vi "CH1603_ONOFF Single Realy.vi"(5 "Loop Read(3)":i32=3, 6 "Relay State":bool, 7 "Device Addr(0x01)":u8=1 format="%02x", 8 "error in (no error)":errorcluster, 9 "Delay Time(200ms)":u32=200, 10 "IO Port No(1~16)":u8=1 format="%02d", 11 "MyIndex":u8) -> (0 "error out":errorcluster, 2 "Result(T:Pass)":bool, 3 "VISA resource name out":refnum<visa-resource-name>)   [LabVIEW 2015]
doc: "Open the device single IO port(1~32),if the IO port no greater than 16,will set the second device IO(device address add 1,the IO port no subtract 16);"
panel:
  out "VISA":refnum<visa-resource-name>
  out "字符串":string
  out "Read String":string
  # "Open Single IO Port"
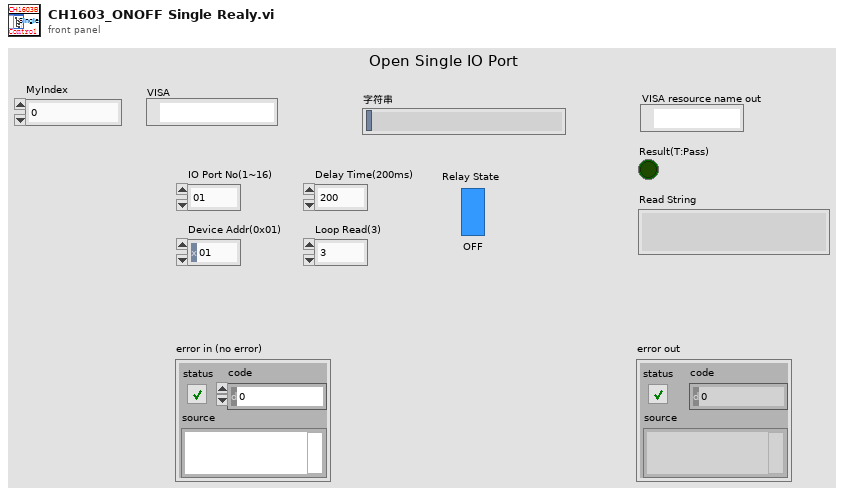
[diagram p1: front panel]
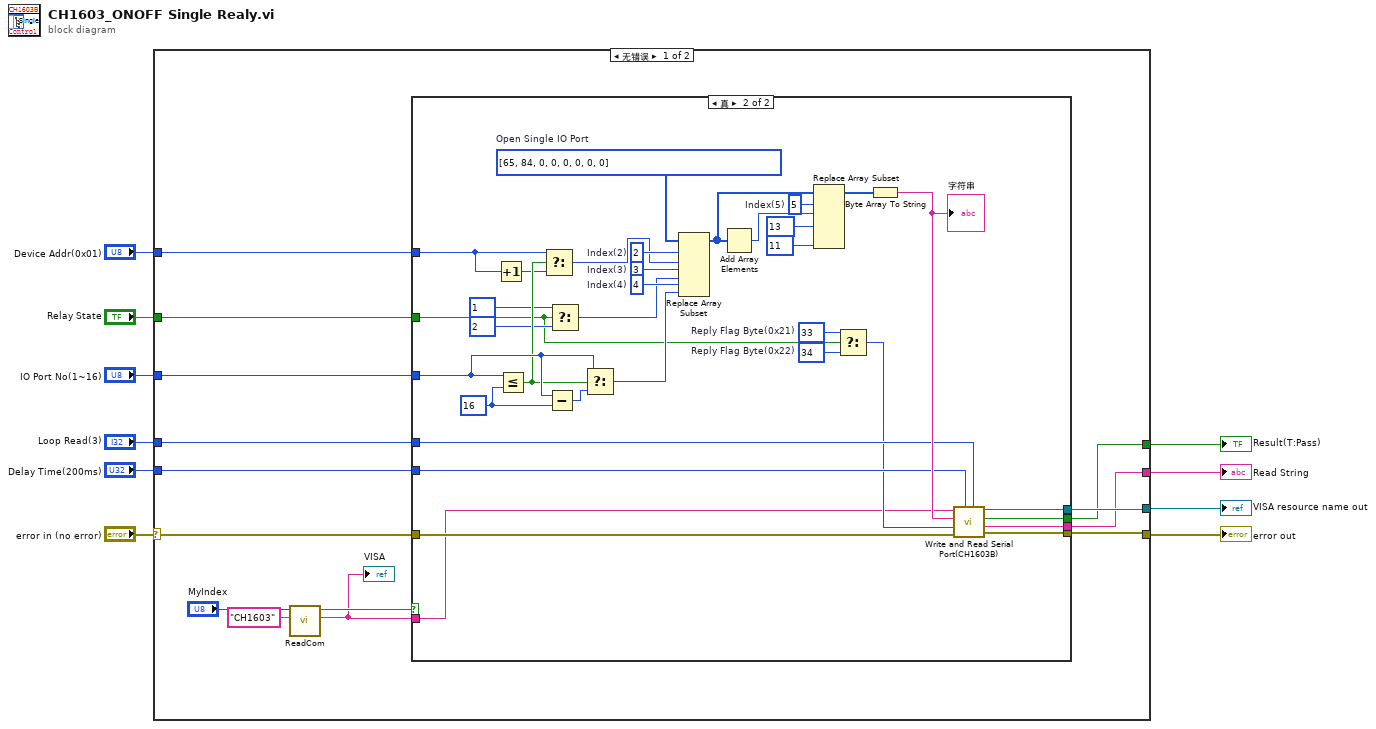
[diagram p0: block diagram]
diagram:
  n1 = case shown="无错误" "error in (no error)" {
    selector: "error in (no error)" -> [w22 w59]
    tunnel: [w19 w59] -> w8
    tunnel: [w18 _] -> w9
    tunnel: "Device Addr(0x01)" -> [w23 _]
    tunnel: "IO Port No(1~16)" -> [w24 _]
    tunnel: "Delay Time(200ms)" -> [w21 _]
    tunnel: [w16 _] -> w4
    tunnel: "Loop Read(3)" -> [w20 _]
    tunnel: [w17 _] -> w2
    tunnel: "Relay State" -> [w15 _]
    frame No Error {
      n2 = call "ReadCom.vi"("仪器名称"="CH1603", "MyIndex"="MyIndex") -> ("COM"=w11:string, "OK?"=w12:bool)  [unwired: 7 in, 1 out]
      "VISA" <- w11
      n3 = case shown="真" w12 {
        tunnel: w24 -> [_ w51]
        tunnel: w23 -> [_ w48]
        tunnel: w22 -> [_ w44]
        tunnel: w21 -> [_ w42]
        tunnel: w20 -> [_ w41]
        tunnel: [_ w40] -> w19
        tunnel: [_ w39] -> w18
        tunnel: [_ w38] -> w17
        tunnel: [_ w37] -> w16
        tunnel: w15 -> [_ w29]
        tunnel: w11 -> [_ w25]
        frame False {
        }
        frame True {
          w27 = u8 34  # Reply Flag Byte(0x22)
          w28 = u8 33  # Reply Flag Byte(0x21)
          w34 = 3  # Index(3)
          w50 = u8 16 ("Device Addr(0x01) 2")
          w56 = 5  # Index(5)
          w35 = 4  # Index(4)
          w57 = 2  # Index(2)
          w58 = u8[] [65, 84, 0, 0, 0, 0, 0, 0]  # Open Single IO Port
          n4 = Increment(x=w48) -> (x+1=w47:u8)
          n5 = Less Or Equal?(x=w51, y=w50) -> (x <= y?=w49:bool)
          n6 = Select(t=w48, s=w49, f=w47) -> (s? t:f=w33:u8)
          n7 = Subtract(x=w51, y=w50) -> (x-y=w52:u8)
          n8 = Select(t=u8 1 ("Device Addr(0x01) 2"), s=w29, f=2 ("Device Addr(0x01) 2")) -> (s? t:f=w30:i32)
          n9 = Select(t=w51, s=w49, f=w52) -> (s? t:f=w36:u8)
          n10 = Replace Array Subset(array=w58, new element #1=w33, index #1=w57, new element #2=w30, index #2=w34, new element #3=w36, index #3=w35) -> (w46:u8[])
          n11 = Add Array Elements(numeric array=w46) -> (sum=w45:u8)
          n12 = Replace Array Subset(array=w46, new element #1=w45, index #1=w56, new element #2=u8 13 ("Device Addr(0x01) 2"), new element #3=u8 11 ("Device Addr(0x01) 2")) -> (w53:u8[])  [unwired: 2 in]
          n13 = Select(t=w28, s=w29, f=w27) -> (s? t:f=w26:u8)
          n14 = Byte Array To String(unsigned byte array=w53) -> (string=w43:string)
          "字符串" <- w43
          n15 = call "Write and Read Serial Port(CH1603B).vi"("Loop Read(3)"=w41, "Delay Time(200ms)"=w42, "error in (no error)"=w44, "Reply Flag Byte"=w26, "Write Command"=w43, "VISA resource name in"=w25) -> ("error out"=w40:errorcluster, "Read String"=w37:string, "Result(T:Pass)"=w38:bool, "VISA resource name out"=w39:refnum<visa-resource-name>)  [unwired: 2 in]
        }
      }
    }
    frame Error {
    }
  }
  "VISA resource name out" <- w9
  "error out" <- w8
  "Read String" <- w4
  "Result(T:Pass)" <- w2
